vi "Add.vi"(0 "reference in":refnum<class "BrowerComposite.lvclass">, 1 "BrowerComponents":refnum<class "BrowerComponent.lvclass">[](array[class]), 5 "error in (no error)":errorcluster) -> (14 "reference out":refnum<class "BrowerComposite.lvclass">, 19 "error out":errorcluster)   [LabVIEW 2015, in "BrowerComposite.lvclass"]
uses:
  BrowerComposite.lvclass
  BrowerComponent/BrowerComponent.lvclass
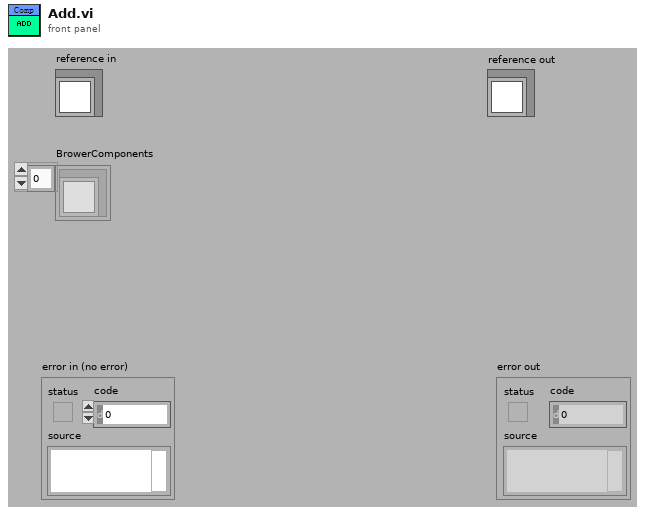
[diagram p1: front panel]
types:
  T1 = typedef "BrowerComposite.lvclass/ObjectAttributes.ctl" = cluster{"BrowerComponents":refnum<class "BrowerComponent.lvclass">[], "BrowerComponentIDs":string[]}
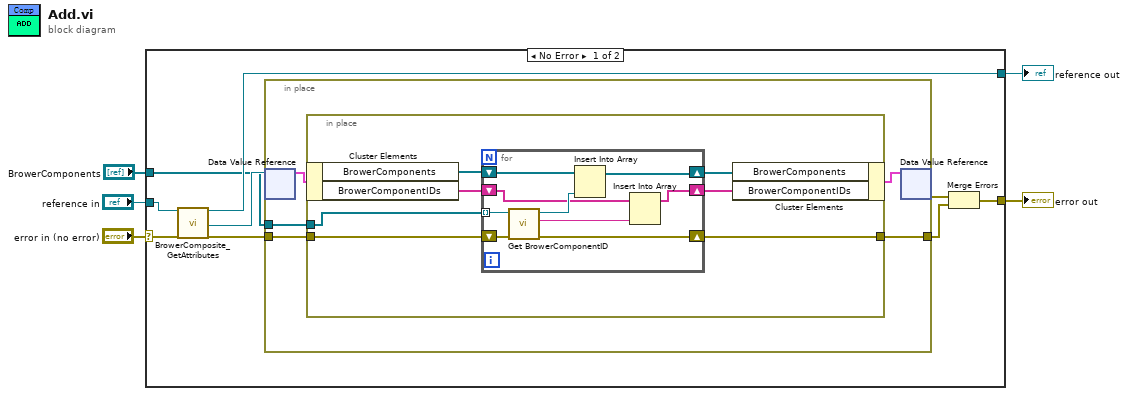
[diagram p0: block diagram]
diagram:
  n1 = case shown="No Error" "error in (no error)" {
    selector: "error in (no error)" -> [w14 w37]
    tunnel: [w12 w37] -> w4
    tunnel: [w11 w36] -> w2
    tunnel: "reference in" -> [w6 w36]
    tunnel: "BrowerComponents" -> [w9 _]
    frame No Error {
      n2 = call "BrowerComposite_GetAttributes.vi"("reference in"=w6, "error in (no error)"=w14) -> ("reference out"=w11:refnum<class "BrowerComposite.lvclass">, "DataRef"=w10:refnum<data-value>, "error out"=w8:errorcluster)  [unwired: 14 in, 1 out]
      n3 = in-place {
        in-place-border: w9 -> [w18]
        in-place-border: w8 -> [w17]
        in-place-border: [w15] -> w7
        n4 = in-place-dvr #1(w10) -> (w19:T1)  [unwired: 1 out]
        n5 = in-place {
          in-place-border: w18 -> [w26]
          in-place-border: w17 -> [w25]
          in-place-border: [w24] -> w15
          n6 = in-place-cluster #2(w19) -> ("BrowerComponents"=w23:refnum<class "BrowerComponent.lvclass">[], "BrowerComponentIDs"=w22:string[])
          n7 = for {
            tunnel: w26 -> [w35] mode=indexing
            shift-right: [w31] -> w24
            shift-left: w25 -> [w34]
            shift-right: [w30] -> w20
            shift-left: w23 -> [w33]
            shift-right: [w27] -> w21
            shift-left: w22 -> [w29]
            n8 = call "Get BrowerComponentID.vi"("error in (no error)"=w34, "BrowerComponent in"=w35) -> ("error out"=w31:errorcluster, "ComponentID"=w28:string, "BrowerComponent out"=w32:refnum<class "BrowerComponent.lvclass">)  [unwired: 7 in]
            n9 = Insert Into Array(array=w33, new element=w32) -> (w30:refnum<class "BrowerComponent.lvclass">[])  [unwired: 1 in]
            n10 = Insert Into Array(array=w29, new element=w28) -> (w27:string[])  [unwired: 1 in]
          }
          n11 = in-place-cluster #2("BrowerComponents"=w20, "BrowerComponentIDs"=w21) -> (w16:T1)
        }
        n12 = in-place-dvr #1(w16) -> (w13:errorcluster)  [unwired: 1 out]
      }
      n13 = Merge Errors(w13, w7) -> (w12:errorcluster)
    }
    frame Error {
    }
  }
  "error out" <- w4
  "reference out" <- w2
